vi "Validate_string.vi"(8 "error in (no error)":errorcluster, 9 "Be verbose (F)":bool, 10 "String data format":string, 11 "String":string) -> (0 "error out":errorcluster, 3 "String Valid":bool)   [LabVIEW 2013]
doc: "Validates string contents using format string. \nFirst 2 digits are minimum length. Make 0 if don't care.\nNext 2 digits are maximum length. Make 99 if don't care.\nEach digit after first 4 length specifiers describe what that digit can be in the string.\n* = must be that char in format string, x means don't care, n means number 0-9,\na mean alpha upper or lower case, r means alpha or number (a/n),\nh means hex digits 0-9, a-f, A-F"
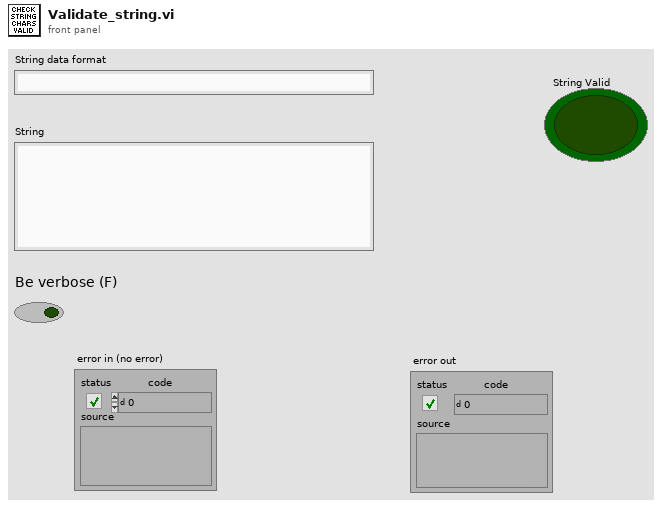
[diagram p1: front panel]
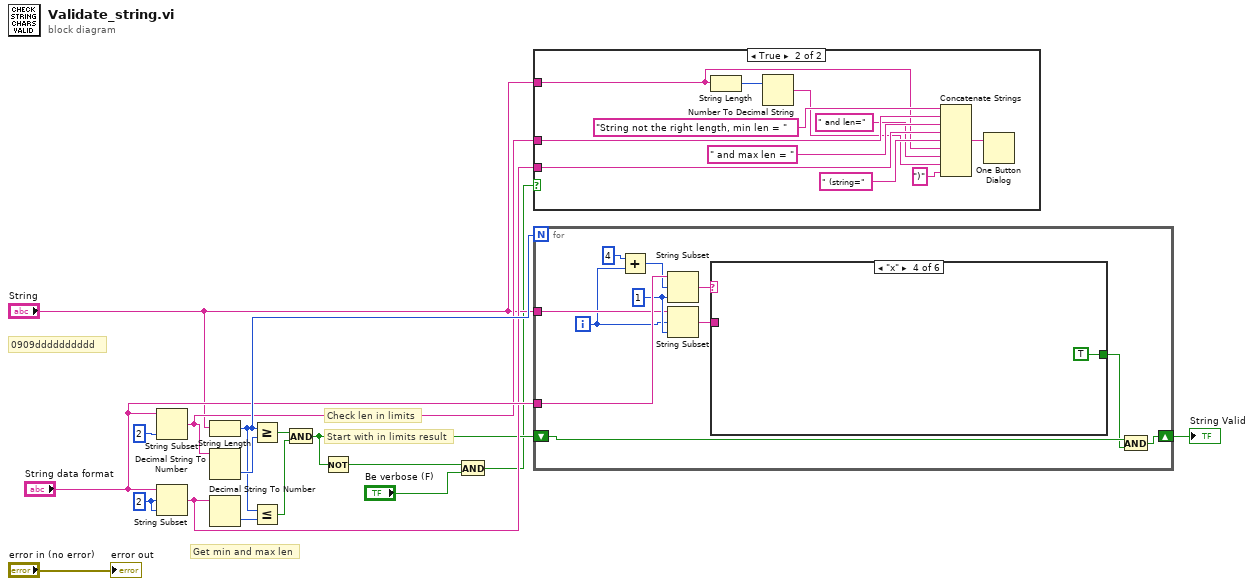
[diagram p0: block diagram]
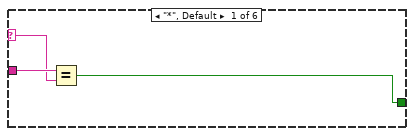
[diagram p3: hidden frame]
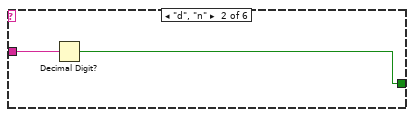
[diagram p4: hidden frame]
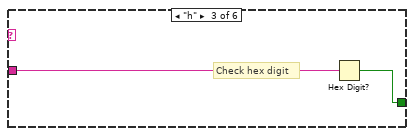
[diagram p5: hidden frame]
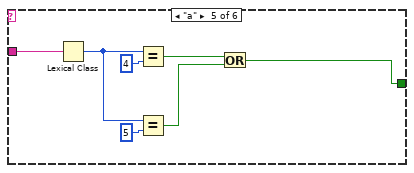
[diagram p6: hidden frame]
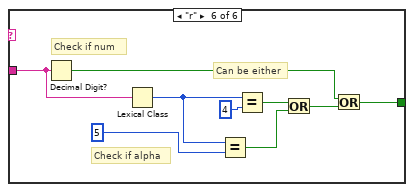
[diagram p7: hidden frame]
diagram:
  w14 = 2 ("offset (0)")
  # "0909dddddddddd"
  # "Start with in limits result"
  # "Check len in limits"
  # "Get min and max len"
  n1 = String Subset(string="String data format", length (rest)=2 ("length (rest)")) -> (substring=w7:string)  [unwired: 1 in]
  n2 = String Subset(string="String data format", offset (0)=w14, length (rest)=w14) -> (substring=w6:string)
  n3 = String Length(string="String") -> (length=w9:i32)
  n4 = Decimal String To Number(string=w7) -> (number=w13:i32)  [unwired: 2 in, 1 out]
  n5 = Decimal String To Number(string=w6) -> (number=w12:i32)  [unwired: 2 in, 1 out]
  n6 = Greater Or Equal?(x=w9, y=w13) -> (x >= y?=w11:bool)
  n7 = Less Or Equal?(x=w9, y=w12) -> (x <= y?=w10:bool)
  n8 = And(x=w11, y=w10) -> (x .and. y?=w4:bool)
  n9 = Not(x=w4) -> (.not. x?=w3:bool)
  n10 = And(x=w3, y="Be verbose (F)") -> (x .and. y?=w1:bool)
  n11 = case shown="True" w1 {
    tunnel: w7 -> [_ w27]
    tunnel: w6 -> [_ w25]
    tunnel: "String" -> [_ w22]
    frame False {
    }
    frame True {
      n12 = String Length(string=w22) -> (length=w21:i32)
      n13 = Number To Decimal String(number=w21) -> (decimal integer string=w20:string)  [unwired: 1 in]
      n14 = Concatenate Strings("String not the right length, min len = " ("message"), w27, " and max len = " ("string"), w25, " (string=" ("string"), w22, " and len=" ("string"), w20, ")" ("string")) -> (w18:string)
      n15 = One Button Dialog(message=w18) -> ()  [unwired: 1 in, 1 out]
    }
  }
  n16 = for {
    N: w9 -> [_]
    tunnel: "String data format" -> [w39]
    tunnel: "String" -> [w35]
    shift-right: [w34] -> w17
    shift-left: w4 -> [w33]
    i -> [w29]
    w37 = 1 ("length (rest)")
    n17 = Add(x=4, y=w29) -> (x+y=w30:i32)
    n18 = String Subset(string=w39, offset (0)=w30, length (rest)=w37) -> (substring=w38:string)
    n19 = String Subset(string=w35, offset (0)=w29, length (rest)=w37) -> (substring=w36:string)
    n20 = case shown="\"x\"" w38 {
      selector: w38 -> [w41 _ _ _ _ _]
      tunnel: w36 -> [w42 w44 w46 _ w53 w58]
      tunnel: [w40 w43 w45 TRUE w48 w55] -> w32
      frame "*", Default {
        n21 = Equal?(x=w42, y=w41) -> (x = y?=w40:bool)
      }
      frame "d", "n" {
        n22 = Decimal Digit?(1:w44) -> (0:w43:bool)
      }
      frame "h" {
        # "Check hex digit"
        n23 = Hex Digit?(1:w46) -> (0:w45:bool)
      }
      frame "x" {
      }
      frame "a" {
        n24 = Lexical Class(1:w53) -> (0:w51:i16)
        n25 = Equal?(x=w51, y=i16 4) -> (x = y?=w49:bool)
        n26 = Equal?(x=w51, y=i16 5) -> (x = y?=w50:bool)
        n27 = Or(x=w49, y=w50) -> (x .or. y?=w48:bool)
      }
      frame "r" {
        # "Can be either"
        # "Check if alpha"
        # "Check if num"
        n28 = Decimal Digit?(1:w58) -> (0:w56:bool)
        n29 = Lexical Class(1:w58) -> (0:w61:i16)
        n30 = Equal?(x=w61, y=i16 5) -> (x = y?=w60:bool)
        n31 = Equal?(x=w61, y=i16 4) -> (x = y?=w59:bool)
        n32 = Or(x=w59, y=w60) -> (x .or. y?=w57:bool)
        n33 = Or(x=w56, y=w57) -> (x .or. y?=w55:bool)
      }
    }
    n34 = And(x=w33, y=w32) -> (x .and. y?=w34:bool)
  }
  "String Valid" <- w17
  "error out" <- "error in (no error)"
